vi "机械手实际坐标去掉负数.vi"(9 "是否自动锁螺丝数组":bool[](array[boolean]), 11 "数组输入":cluster{"X":dbl, "Y":dbl}[](array[cluster])) -> (1 "自动锁螺丝的点位示意图坐标":cluster{dbl, dbl}[](array[cluster]), 3 "所有锁螺丝的点位示意图坐标(包括不自动锁的)":cluster{"X":dbl, "Y":dbl}[](array[cluster]))   [LabVIEW 2014]
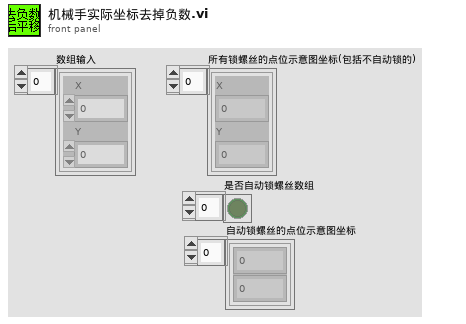
[diagram p1: front panel]
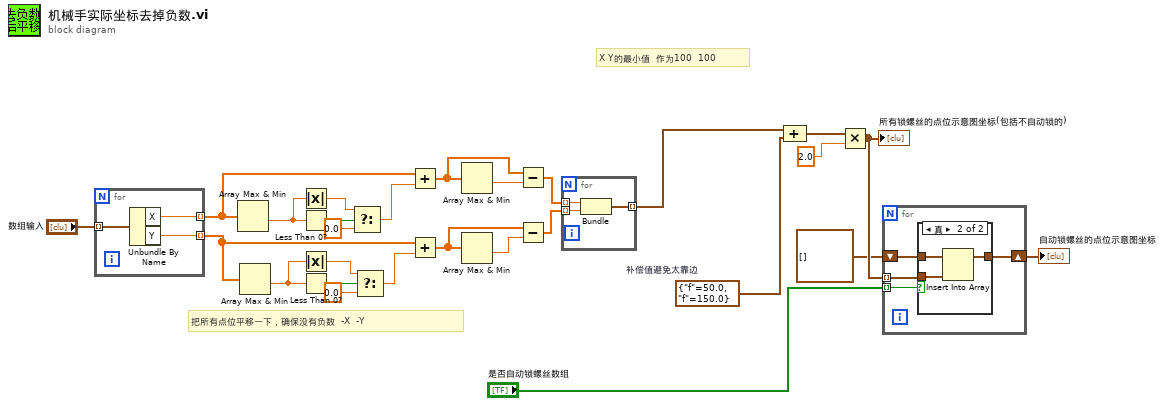
[diagram p0: block diagram]
diagram:
  w19 = cluster{"f":dbl, "f":dbl} {"f"=50.0, "f"=150.0}  # 补偿值避免太靠边
  # "X Y的最小值  作为100  100"
  # "把所有点位平移一下，确保没有负数  -X  -Y"
  n1 = for {
    tunnel: "数组输入" -> [w30] mode=indexing
    tunnel: [w29] -> w16 mode=indexing
    tunnel: [w28] -> w14 mode=indexing
    n2 = Unbundle By Name(w30) -> ("X"=w29:dbl, "Y"=w28:dbl)
  }
  n3 = Array Max & Min(array=w16) -> (min value=w25:dbl)  [unwired: 3 out]
  n4 = Array Max & Min(array=w14) -> (min value=w23:dbl)  [unwired: 3 out]
  n5 = Absolute Value(x=w25) -> (abs(x)=w24:dbl)
  n6 = Less Than 0?(x=w25) -> (x < 0?=w27:bool)
  n7 = Absolute Value(x=w23) -> (abs(x)=w22:dbl)
  n8 = Less Than 0?(x=w23) -> (x < 0?=w26:bool)
  n9 = Select(t=w24, s=w27, f=0.0) -> (s? t:f=w15:dbl)
  n10 = Select(t=w22, s=w26, f=0.0) -> (s? t:f=w13:dbl)
  n11 = Add(x=w16, y=w15) -> (x+y=w12:dbl[])
  n12 = Add(x=w14, y=w13) -> (x+y=w10:dbl[])
  n13 = Array Max & Min(array=w12) -> (min value=w11:dbl)  [unwired: 3 out]
  n14 = Array Max & Min(array=w10) -> (min value=w9:dbl)  [unwired: 3 out]
  n15 = Subtract(x=w12, y=w11) -> (x-y=w8:dbl[])
  n16 = Subtract(x=w10, y=w9) -> (x-y=w7:dbl[])
  n17 = for {
    tunnel: w8 -> [w33] mode=indexing
    tunnel: w7 -> [w32] mode=indexing
    tunnel: [w31] -> w5 mode=indexing
    n18 = Bundle(w33, w32) -> (w31:cluster{dbl, dbl})  [unwired: 1 in]
  }
  n19 = Compound Arithmetic op=ADD(w5, w19) -> (w18:cluster{dbl, dbl}[])
  n20 = Multiply(x=w18, y=2.0 ("f")) -> (x*y=w4:cluster{dbl, dbl}[])
  "所有锁螺丝的点位示意图坐标(包括不自动锁的)" <- w4
  n21 = for {
    tunnel: w4 -> [w34] mode=indexing
    tunnel: "是否自动锁螺丝数组" -> [w37] mode=indexing
    shift-right: [w36] -> w1
    shift-left: cluster{dbl, dbl}[] [] -> [w35]
    n22 = case shown="真" w37 {
      tunnel: w34 -> [_ w41]
      tunnel: [w38 w40] -> w36
      tunnel: w35 -> [w38 w39]
      frame False {
      }
      frame True {
        n23 = Insert Into Array(array=w39, new element=w41) -> (w40:cluster{dbl, dbl}[])  [unwired: 1 in]
      }
    }
  }
  "自动锁螺丝的点位示意图坐标" <- w1
